vi "Make pulse data.vi"(0 "phases":i32=3 caption="Phases", 1 "pulsereps":i32=2 caption="Repetitions", 3 "randomize":bool=TRUE, 5 "pulsedir":enum16{"Left", "Right", "Both"}(ring)=enum."Both" caption="Direction", 7 "sinfreq":dbl=1.5 caption="sinefreq", 9 "Amplitudes":dbl[](array[numeric])=[5.0], 11 "Durations":dbl[](array[numeric])=[0.2], 12 "pre cycles":dbl=10.0 caption="Pre cycles", 13 "post cycles":dbl=10.0 caption="Post cycles", 14 "cyclesperpulse":dbl=10.0 caption="Cycles per pulse") -> (4 "pulse data":T1, 6 "totaltime":dbl caption="Total time")   [LabVIEW 2013]
uses:
  Pulse data.ctl
  <vilib>/gmath/statdist.llb/Random Permutation.vi
  <vilib>/gmath/NI_Gmath.lvlib
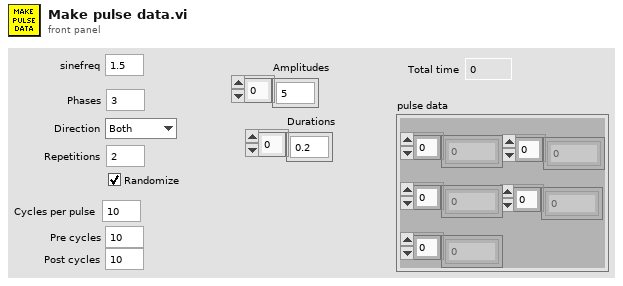
[diagram p1: front panel]
types:
  T1 = typedef "Pulse data.ctl" = cluster{"time":dbl[], "phase":dbl[], "dir/phase2":dbl[], "amplitude":dbl[], "duration":dbl[]}
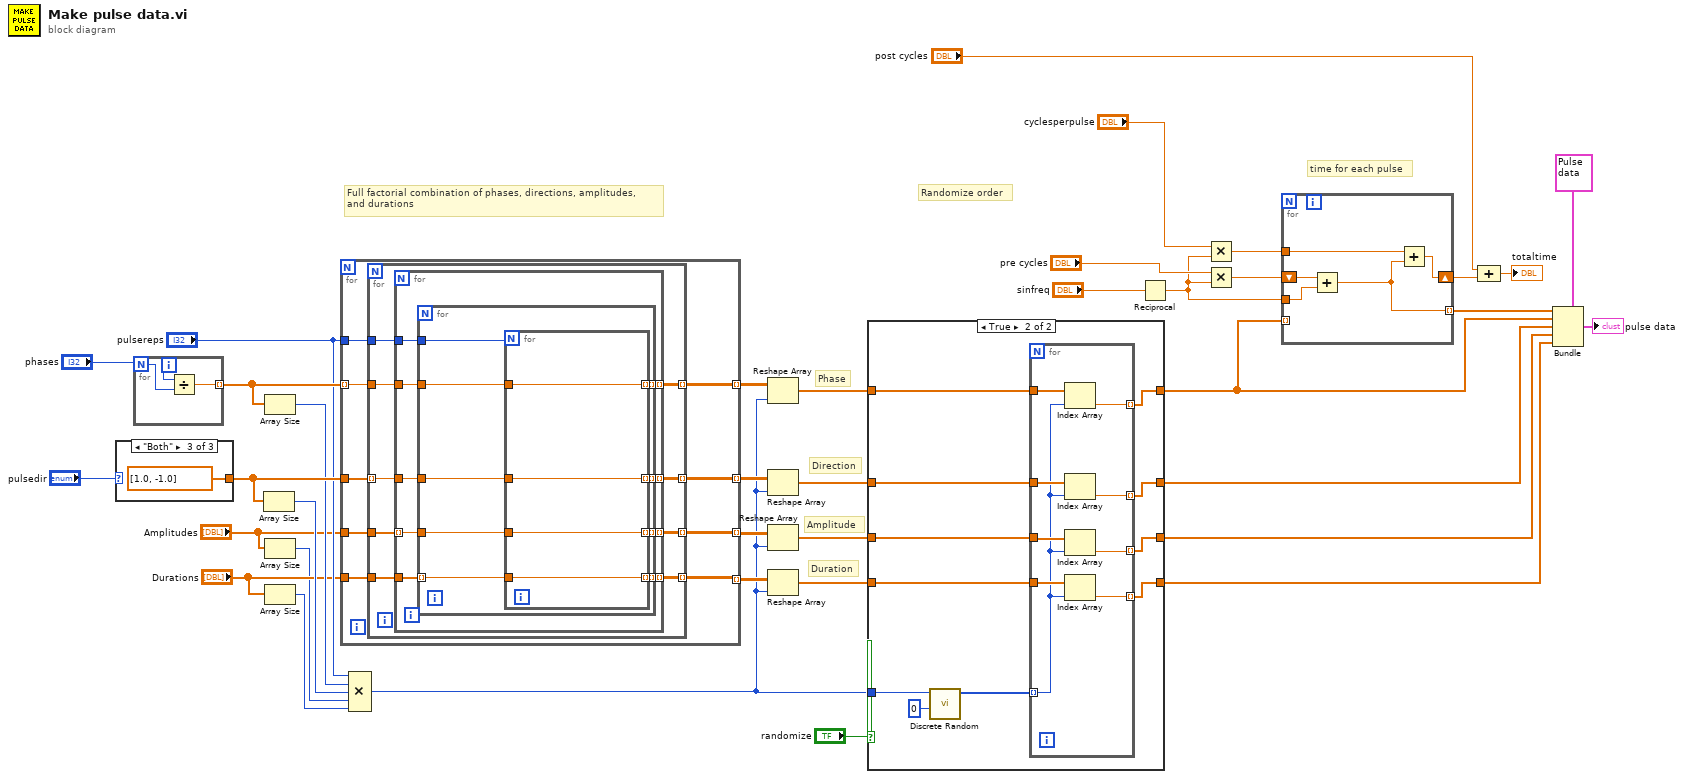
[diagram p0: block diagram]
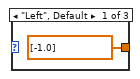
[diagram p3: hidden frame]
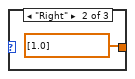
[diagram p4: hidden frame]
diagram:
  # "time for each pulse"
  # "Duration"
  # "Amplitude"
  # "Direction"
  # "Phase"
  # "Randomize order"
  # "Full factorial combination of phases, directions, amplitudes,\nand durations"
  n1 = case shown="\"Both\"" "pulsedir" {
    tunnel: [dbl[] [-1.0] dbl[] [1.0] dbl[] [1.0, -1.0]] -> w33
    frame "Left", Default {
    }
    frame "Right" {
    }
    frame "Both" {
    }
  }
  n2 = for {
    N: "phases" -> [w43]
    tunnel: [w41] -> w34 mode=indexing
    i -> [w42]
    n3 = Divide(x=w42, y=w43) -> (x/y=w41:dbl)
  }
  n4 = Array Size(array=w33) -> (size(s)=w32:i32)
  n5 = Array Size(array=w34) -> (size(s)=w31:i32)
  n6 = Array Size(array="Amplitudes") -> (size(s)=w23:i32)
  n7 = Array Size(array="Durations") -> (size(s)=w22:i32)
  n8 = for {
    tunnel: w34 -> [w50] mode=indexing
    tunnel: w33 -> [w52]
    tunnel: "pulsereps" -> [w51]
    tunnel: [w49] -> w35 mode=indexing
    tunnel: [w48] -> w29 mode=indexing
    tunnel: "Amplitudes" -> [w47]
    tunnel: [w46] -> w21 mode=indexing
    tunnel: "Durations" -> [w45]
    tunnel: [w44] -> w20 mode=indexing
    n9 = for {
      tunnel: w52 -> [w59] mode=indexing
      tunnel: w51 -> [w61]
      tunnel: w50 -> [w60]
      tunnel: [w58] -> w49 mode=indexing
      tunnel: [w57] -> w48 mode=indexing
      tunnel: w47 -> [w56]
      tunnel: [w55] -> w46 mode=indexing
      tunnel: w45 -> [w54]
      tunnel: [w53] -> w44 mode=indexing
      n10 = for {
        tunnel: w61 -> [w70]
        tunnel: w60 -> [w69]
        tunnel: w59 -> [w68]
        tunnel: [w67] -> w58 mode=indexing
        tunnel: [w66] -> w57 mode=indexing
        tunnel: w56 -> [w65] mode=indexing
        tunnel: [w64] -> w55 mode=indexing
        tunnel: w54 -> [w63]
        tunnel: [w62] -> w53 mode=indexing
        n11 = for {
          tunnel: w70 -> [w79]
          tunnel: w69 -> [w78]
          tunnel: w68 -> [w77]
          tunnel: [w76] -> w67 mode=indexing
          tunnel: [w75] -> w66 mode=indexing
          tunnel: w65 -> [w74]
          tunnel: [w73] -> w64 mode=indexing
          tunnel: w63 -> [w72] mode=indexing
          tunnel: [w71] -> w62 mode=indexing
          n12 = for {
            N: w79 -> [_]
            tunnel: w78 -> [w83]
            tunnel: w77 -> [w82]
            tunnel: [w83] -> w76 mode=indexing
            tunnel: [w82] -> w75 mode=indexing
            tunnel: w74 -> [w80]
            tunnel: [w81] -> w73 mode=indexing
            tunnel: w72 -> [w81]
            tunnel: [w80] -> w71 mode=indexing
          }
        }
      }
    }
  }
  n13 = Compound Arithmetic op=MULTIPLY("pulsereps", w31, w32, w23, w22) -> (w19:i32)
  n14 = Reshape Array(w35, w19) -> (w27:dbl[])
  n15 = Reshape Array(w29, w19) -> (w26:dbl[])
  n16 = Reshape Array(w20, w19) -> (w18:dbl[])
  n17 = Reshape Array(w21, w19) -> (w17:dbl[])
  n18 = case shown="True" "randomize" {
    tunnel: w19 -> [_ w97]
    tunnel: w27 -> [w87 w96]
    tunnel: w26 -> [w86 w95]
    tunnel: [w87 w92] -> w2
    tunnel: [w86 w93] -> w15
    tunnel: w18 -> [w85 w91]
    tunnel: w17 -> [w84 w90]
    tunnel: [w85 w89] -> w14
    tunnel: [w84 w88] -> w13
    frame False {
    }
    frame True {
      n19 = call-poly <vilib>:"Discrete Random.vi"("start"=0, "N"=w97) -> ("random permutation"=w94:i32[])  [unwired: 8 in, 1 out]
      n20 = for {
        tunnel: w96 -> [w107]
        tunnel: w95 -> [w106]
        tunnel: w94 -> [w101] mode=indexing
        tunnel: [w105] -> w92 mode=indexing
        tunnel: [w104] -> w93 mode=indexing
        tunnel: w91 -> [w102]
        tunnel: w90 -> [w103]
        tunnel: [w100] -> w89 mode=indexing
        tunnel: [w99] -> w88 mode=indexing
        n21 = Index Array(array=w107, index=w101) -> (element=w105:dbl)
        n22 = Index Array(array=w106, index=w101) -> (element=w104:dbl)
        n23 = Index Array(array=w102, index=w101) -> (element=w100:dbl)
        n24 = Index Array(array=w103, index=w101) -> (element=w99:dbl)
      }
    }
  }
  n25 = Reciprocal(x="sinfreq") -> (1/x=w1:dbl)
  n26 = Multiply(x="cyclesperpulse", y=w1) -> (x*y=w6:dbl)
  n27 = Multiply(x="pre cycles", y=w1) -> (x*y=w4:dbl)
  n28 = for {
    tunnel: w6 -> [w112]
    tunnel: [w109] -> w16 mode=indexing
    shift-right: [w111] -> w3
    shift-left: w4 -> [w110]
    tunnel: w2 -> [_] mode=indexing
    tunnel: w1 -> [w108]
    n29 = Add(x=w110, y=w108) -> (x+y=w109:dbl)
    n30 = Add(x=w112, y=w109) -> (x+y=w111:dbl)
  }
  n31 = Compound Arithmetic op=ADD("post cycles", w3) -> (→"totaltime":dbl)
  n32 = Bundle(cluster=T1 {"time"=[0.2222222222222222, 6.888888888888888, 13.333333333333332, 20.22222222222222, 26.666666666666664, 33.77777777777777, 40.44444444444444, 46.666666666666664, 53.77777777777777, 59.99999999999999, 66.88888888888889, 73.77777777777777], "phase"=[0.3333333333333333, 0.3333333333333333, 0.0, 0.3333333333333333, 0.0, 0.6666666666666666, 0.6666666666666666, 0.0, 0.6666666666666666, 0.0, 0.3333333333333333, 0.6666666666666666], "dir/phase2"=[1.0, -1.0, -1.0, 1.0, 1.0, -1.0, -1.0, -1.0, 1.0, 1.0, -1.0, 1.0], "amplitude"=[5.0, 5.0, 5.0, 5.0, 5.0, 5.0, 5.0, 5.0, 5.0, 5.0, 5.0, 5.0], "duration"=[0.2, 0.2, 0.2, 0.2, 0.2, 0.2, 0.2, 0.2, 0.2, 0.2, 0.2, 0.2]} ("pulse data 2"), "time"=w16, "phase"=w2, "dir/phase2"=w15, "amplitude"=w14, "duration"=w13) -> (→"pulse data":T1)
